vi "Driver - DTACQ - Get List of Commands.vi"(8 "error in":errorcluster, 11 "DTACQ Connection Data In":T1={"Description"="", "Address"="", "Port"=0, "timeout (ms)"=5000, "Termination Character"="\n", "TCP Connection Reference"=refnum, "Open Connection"=FALSE}) -> (0 "error out":errorcluster, 2 "Commands":string[](array[string]), 3 "DTACQ Connection Data Out":T1={"Description"="", "Address"="", "Port"=0, "timeout (ms)"=5000, "Termination Character"="\n", "TCP Connection Reference"=refnum, "Open Connection"=FALSE})   [LabVIEW 2017, in "Communications Library.lvlib"]
doc: "Runs the help command and retrieves the response.\nEach command is outputted as an element of the command array.\nThe commands are ordered in the same order in which they are read from the DTACQ device."
uses:
  Communications Library.lvlib
  Typedefs/DTACQ Connection Data--Cluster.ctl
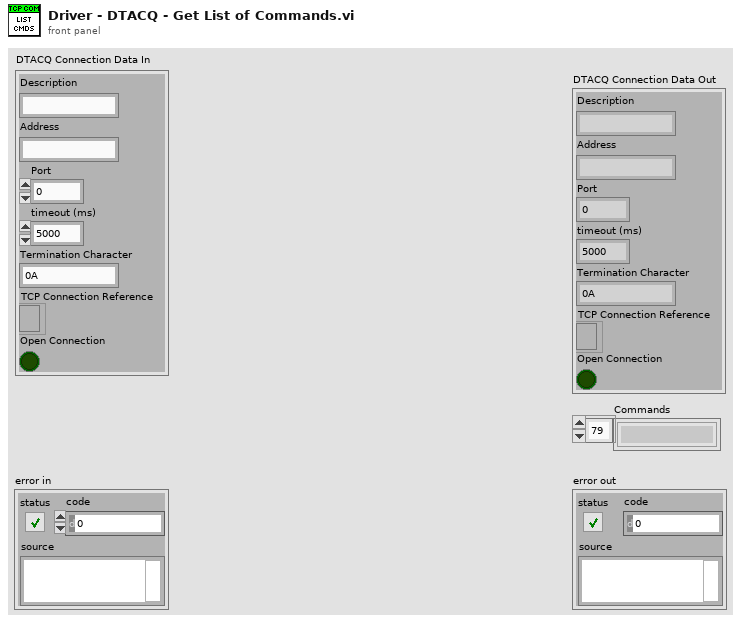
[diagram p1: front panel]
types:
  T1 = typedef "Communications Library.lvlib/DTACQ Connection Data--Cluster.ctl" = cluster{"Description":string, "Address":string, "Port":u16, "timeout (ms)":i32, "Termination Character":string, "TCP Connection Reference":refnum<k5>, "Open Connection":bool}
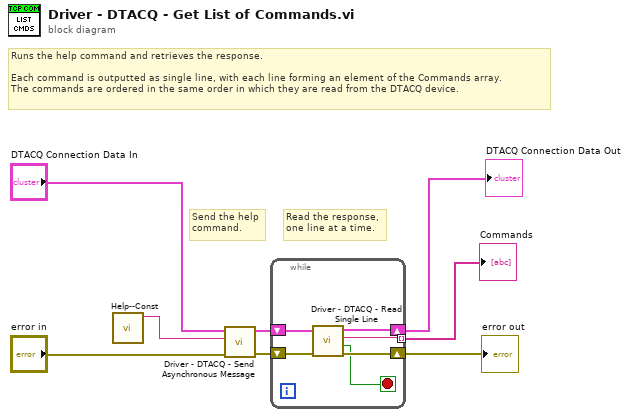
[diagram p0: block diagram]
diagram:
  # "Read the response,\none line at a time."
  # "Send the help\ncommand."
  # "Runs the help command and retrieves the response.\n\nEach command is outputted as single line, with each line forming an element of the Commands array.\nThe commands are ordered in the same order in which they are read from the DTACQ device."
  n1 = call "Help--Const.vi"() -> ("Help Command"=w6:string)  [unwired: 11 in]
  n2 = call "Driver - DTACQ - Send Asynchronous Message.vi"("error in"="error in", "Message to Send"=w6, "DTACQ Connection Data In"="DTACQ Connection Data In") -> ("error out"=w5:errorcluster, "DTACQ Connection Data Out"=w4:T1)  [unwired: 7 in]
  n3 = while {
    shift-right: [w10] -> w1
    shift-left: w4 -> [w13]
    shift-right: [w12] -> w3
    shift-left: w5 -> [w14]
    tunnel: [w9] -> w2 mode=indexing
    stop <- w11 stop-if-true
    n4 = call "Driver - DTACQ - Read Single Line.vi"("error in"=w14, "DTACQ Connection Data In"=w13) -> ("error out"=w12:errorcluster, "Timed Out"=w11:bool, "Read String"=w9:string, "DTACQ Connection Data Out"=w10:T1)  [unwired: 6 in]
  }
  "error out" <- w3
  "Commands" <- w2
  "DTACQ Connection Data Out" <- w1
